vi "Calc Freq.vi"(10 "Threshold":dbl=2.0, 11 "waveform":waveform(dbl)) -> (3 "Freq":dbl)   [LabVIEW 2017]
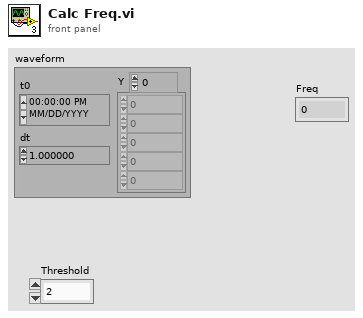
[diagram p1: front panel]
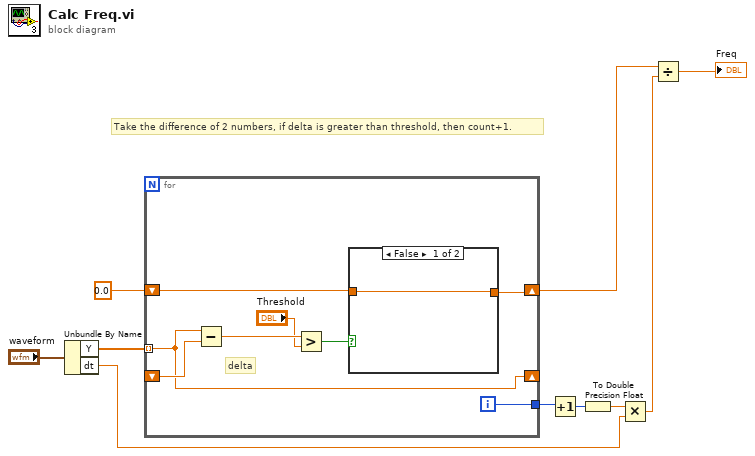
[diagram p0: block diagram]
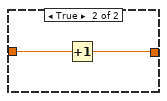
[diagram p2: hidden frame]
diagram:
  # "Take the difference of 2 numbers, if delta is greater than threshold, then count+1."
  n1 = Unbundle By Name("waveform") -> ("Y"=w7:dbl[], "dt"=w2:dbl)
  n2 = for {
    shift-right: [w15] -> _
    shift-left: _ -> [w16]
    shift-right: [w17] -> w9
    shift-left: 0.0 -> [w18]
    tunnel: w7 -> [w15] mode=indexing
    tunnel: [w14] -> w6
    i -> [w14]
    # "delta"
    n3 = Subtract(x=w15, y=w16) -> (x-y=w13:dbl)
    n4 = Greater?(x=w13, y="Threshold") -> (0:w12:bool)
    n5 = case shown="False" w12 {
      tunnel: w18 -> [w19 w21]
      tunnel: [w19 w20] -> w17
      frame False {
      }
      frame True {
        n6 = Increment(x=w21) -> (x+1=w20:dbl)
      }
    }
  }
  n7 = Increment(x=w6) -> (x+1=w5:i32)
  n8 = To Double Precision Float(number=w5) -> (double precision float=w4:dbl)
  n9 = Multiply(x=w4, y=w2) -> (x*y=w3:dbl)
  n10 = Divide(x=w9, y=w3) -> (x/y=→"Freq":dbl)
